vi "4DOF_Serial_Write_Read_Event_xbox_Polling.vi"() -> ()   [LabVIEW 2023]
uses:
  <vilib>/MakerHub/Xbox-One-Controller/Private/Type Defs/Indicators/Controller.ctl
  <vilib>/MakerHub/Xbox-One-Controller/Private/Type Defs/Indicators/A.ctl
  <vilib>/MakerHub/Xbox-One-Controller/Private/Type Defs/Indicators/B.ctl
  <vilib>/MakerHub/Xbox-One-Controller/Private/Type Defs/Indicators/X.ctl
  <vilib>/MakerHub/Xbox-One-Controller/Private/Type Defs/Indicators/Y.ctl
  <vilib>/MakerHub/Xbox-One-Controller/Private/Type Defs/Indicators/Left Bumper.ctl
  <vilib>/MakerHub/Xbox-One-Controller/Private/Type Defs/Indicators/Right Bumper.ctl
  <vilib>/MakerHub/Xbox-One-Controller/Private/Type Defs/Indicators/View.ctl
  <vilib>/MakerHub/Xbox-One-Controller/Private/Type Defs/Indicators/Menu.ctl
  <vilib>/MakerHub/Xbox-One-Controller/Private/Type Defs/Indicators/Thumbstick_Analog.ctl
  <vilib>/MakerHub/Xbox-One-Controller/Private/Type Defs/Indicators/Slider.ctl
  <vilib>/MakerHub/Xbox-One-Controller/Private/Type Defs/Indicators/DPad.ctl
  <vilib>/MakerHub/Xbox-One-Controller/Public/Open First Controller.vi
  <vilib>/Instr/_visa.llb/VISA Configure Serial Port (Instr).vi
  <vilib>/MakerHub/Xbox-One-Controller/LMH-Xbox-One-Controller.lvlib
panel:
  in  "?":bool
  in  "?":bool
  out "length":i32
  out "IK Cartesian \nCordinates (mm)\nLast Sent":string
  in  "Enter IK (X/Y/Z)":string[](array[string])
  in  "Refresh Buffer":bool
  out "X Axis Right":i32 format="%#.0f"
  out "Y Axis Left":i32
  out "Error Out":errorcluster
  in  "byte count\nRead":u32=80
  out "Serial Buffer (Read)":string
  in  "Left Stick":u32(slide)=50 scale=0.0..100.0
  out "Loop Count":i32
  out "Panel Controls\nActive":bool
  in  "Right Bumper":T1 caption="Blank Button"
  in  "Left Bumper":T2 caption="Blank Button"
  in  "Jog\nS_Joint_State\nVia Manual Jog":T3 caption="Blank Button"
  in  "Jog\nS_Main_System_State":T4 caption="Blank Button"
  in  "Home J4":T5 caption="Blank Button"
  in  "Home J2":T6 caption="Blank Button"
  in  "Home J3":T7 caption="Blank Button"
  in  "Home J1":T8 caption="Blank Button"
  in  "Right Stick":u32(slide)=50 scale=0.1..100.0
  in  "Panel Buttons / Xbox Buttons":bool
  out "Controller":T9={"A Button"=FALSE, "B Button"=FALSE, "X Button"=FALSE, "Y Button"=FALSE, "Left Bumper"=FALSE, "Right Bumper"=FALSE, "View Button"=FALSE, "Menu Button"=FALSE, "Left Stick"={[], []}, "Right Stick"={[], []}, "Trigger"=0, "D-Pad"=5} {"Trigger" scale=32767.0..-32768.0}
  out "error out":errorcluster
  in  "error in (no error)":errorcluster
  in  "Loop Timer ms":u32=5 min=10
  out "Concatenated \nString For Transmission":string
  in  "VISA resource name":refnum<visa-resource-name>="COM8"
  out "byte count \nSent":u32
  out "Controller Outputs\nActive":bool
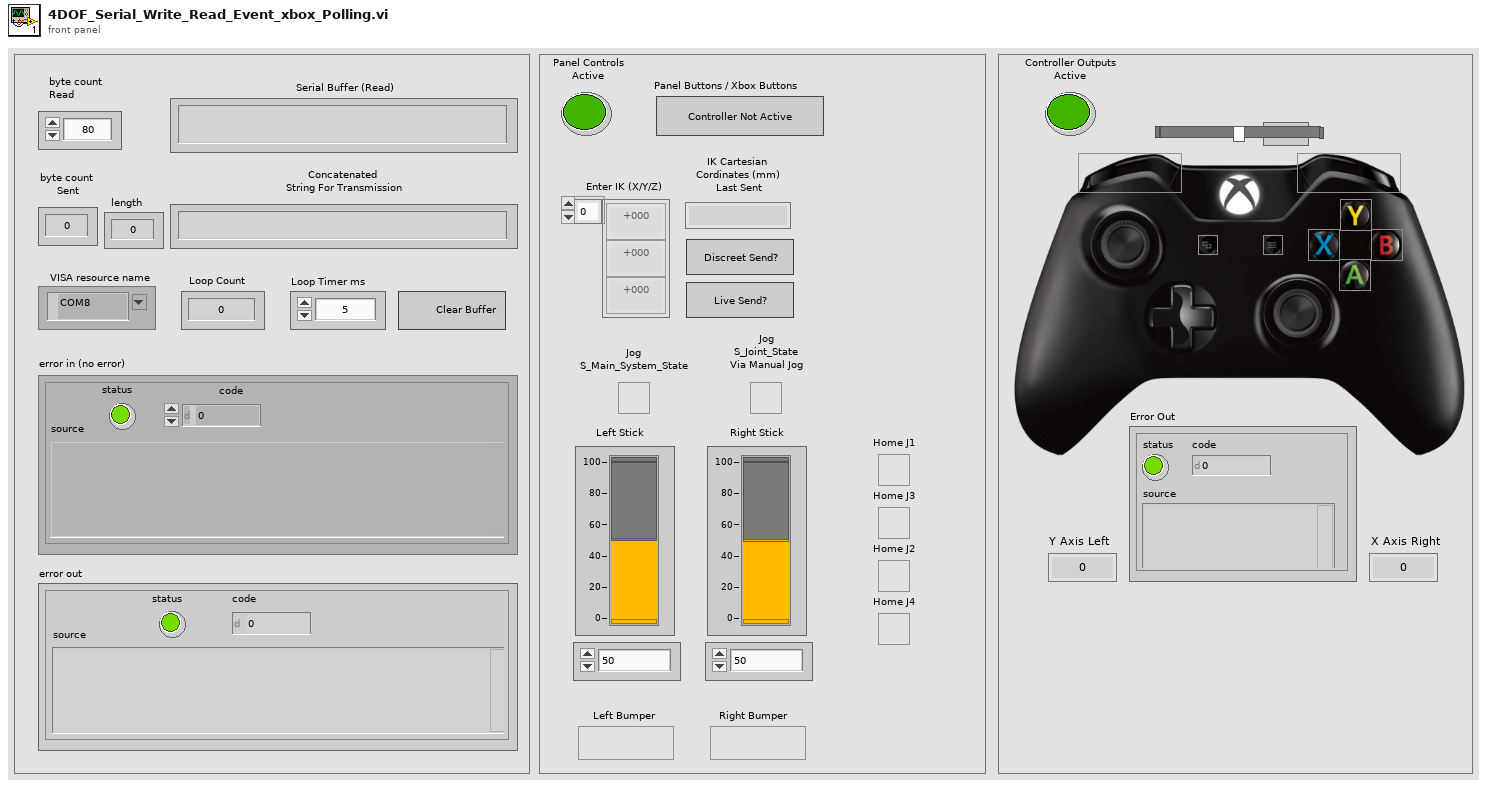
[diagram p1: front panel]
types:
  T1 = typedef "LMH-Xbox-One-Controller.lvlib/Right Bumper.ctl" = bool
  T2 = typedef "LMH-Xbox-One-Controller.lvlib/Left Bumper.ctl" = bool
  T3 = typedef "LMH-Xbox-One-Controller.lvlib/Menu.ctl" = bool
  T4 = typedef "LMH-Xbox-One-Controller.lvlib/View.ctl" = bool
  T5 = typedef "LMH-Xbox-One-Controller.lvlib/Y.ctl" = bool
  T6 = typedef "LMH-Xbox-One-Controller.lvlib/X.ctl" = bool
  T7 = typedef "LMH-Xbox-One-Controller.lvlib/B.ctl" = bool
  T8 = typedef "LMH-Xbox-One-Controller.lvlib/A.ctl" = bool
  T9 = typedef "LMH-Xbox-One-Controller.lvlib/Controller.ctl" = cluster{"A Button":T8, "B Button":T7, "X Button":T6, "Y Button":T5, "Left Bumper":T2, "Right Bumper":T1, "View Button":T4, "Menu Button":T3, "Left Stick":T10, "Right Stick":T10, "Trigger":T11, "D-Pad":T12}
  T10 = typedef "LMH-Xbox-One-Controller.lvlib/Thumbstick_Analog.ctl" = cluster{i32[], i32[]}
  T11 = typedef "LMH-Xbox-One-Controller.lvlib/Slider.ctl" = i32
  T12 = typedef "LMH-Xbox-One-Controller.lvlib/DPad.ctl" = u16
  T13 = typedef "LMH-Xbox-One-Controller.lvlib/Xbox One Controller Ref.ctl" = cluster{"Controller Ref":refnum<k1>, "Event Refnum":refnum<event-registration>, "Worker Ref":refnum<vi>}
  T14 = typedef "LMH-Xbox-One-Controller.lvlib/All Axis Data.ctl" = cluster{"Left Stick":cluster{"X Axis":i32, "Y Axis":i32}, "Right Stick":cluster{"X Axis":i32, "Y Axis":i32}, "Triggers":i32, "D-Pad":T15}
  T15 = typedef "LMH-Xbox-One-Controller.lvlib/DPad Enum.ctl" = enum16{"Idle", "Up", "Up / Right", "Right", "Down / Right", "Down", "Down / Left", "Left", "Up / Left"}
  T16 = typedef "LMH-Xbox-One-Controller.lvlib/All Buttons Visual.ctl" = cluster{"A":T8, "B":T7, "X":T6, "Y":T5, "Left Bumper":T2, "Right Bumper":T1, "View Button":T4, "Menu Button":T3, "Left Stick":T17, "Right Stick":T17}
  T17 = typedef "LMH-Xbox-One-Controller.lvlib/Thumbstick.ctl" = bool
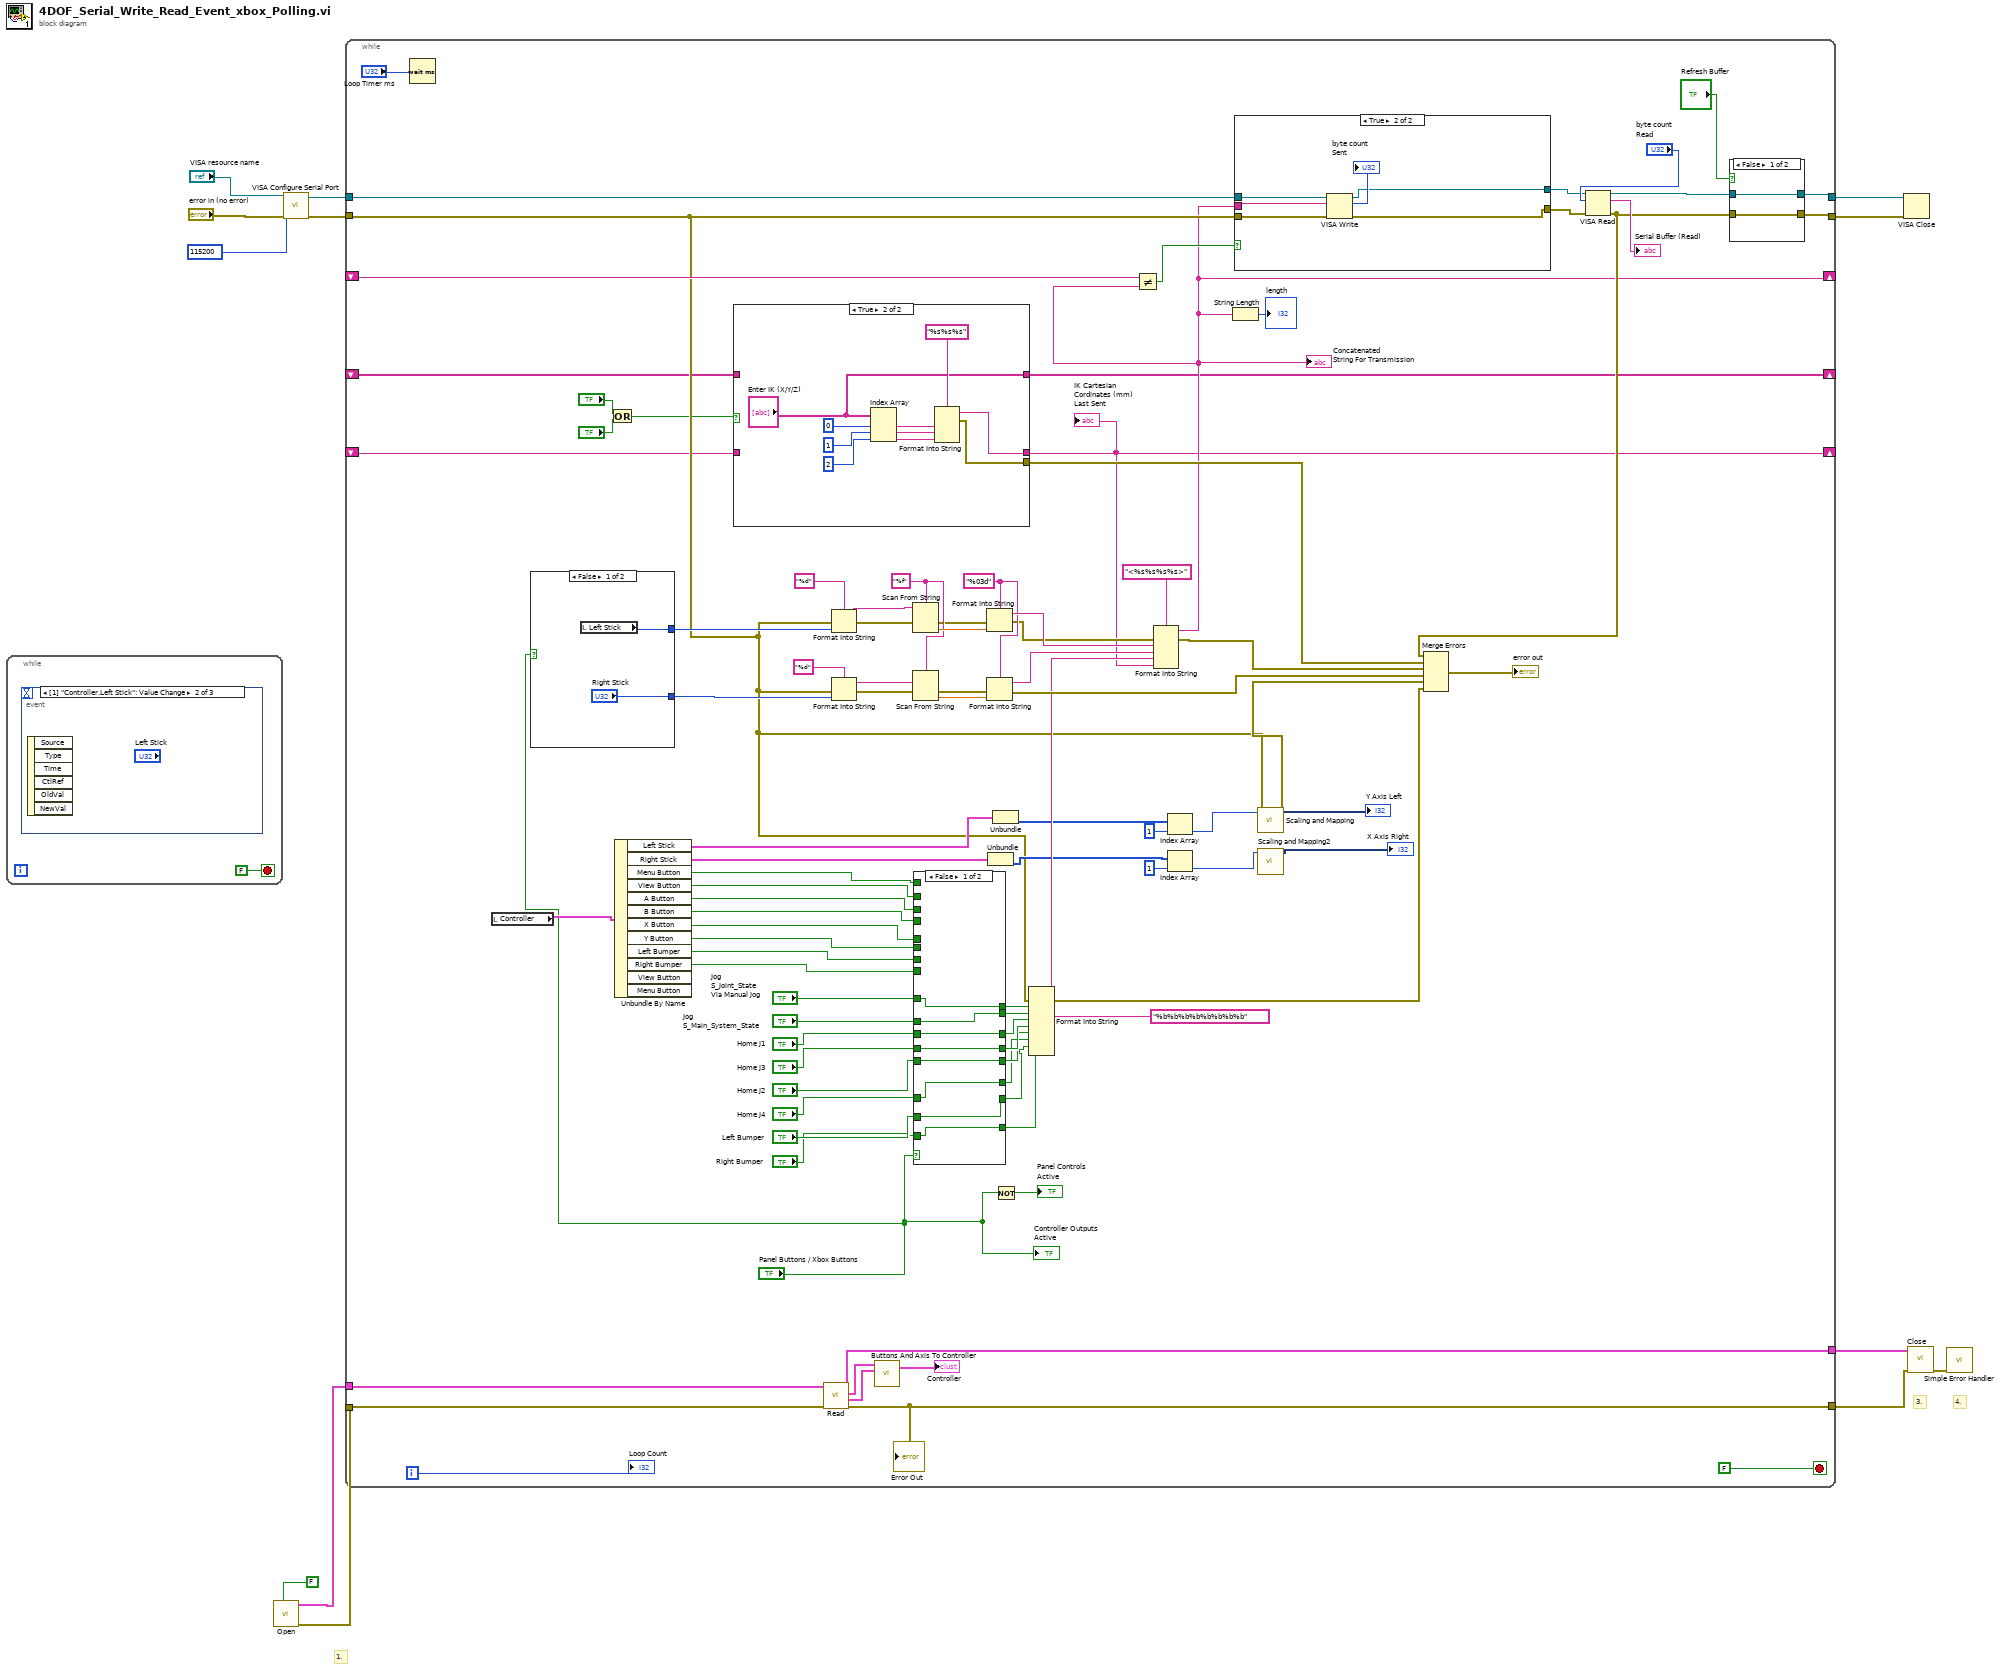
[diagram p0: block diagram]
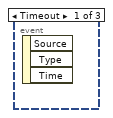
[diagram p2: hidden frame]
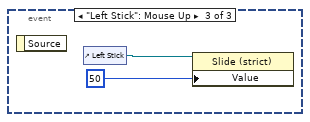
[diagram p3: hidden frame]
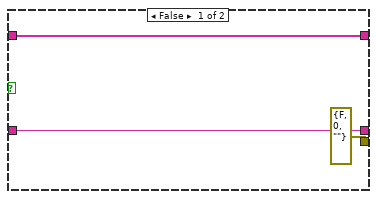
[diagram p4: hidden frame]
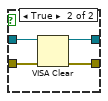
[diagram p5: hidden frame]
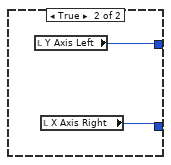
[diagram p6: hidden frame]
diagram:
  # "4."
  # "3."
  # "1."
  n1 = while {
    stop <- FALSE stop-if-true
    n2 = event shown="[1] \"Controller.Left Stick\": Value Change" {
      selector: _ -> [_ _ _]
      dyn-events: _ -> [_ _ _]
      timeout: _ -> [_ _ _]
      event Timeout {
        n3 = event-data() -> ()  [unwired: 1 in, 3 out]
      }
      event Value Change {
        n4 = event-data() -> ()  [unwired: 1 in, 6 out]
      }
      event "Left Stick": Mouse Up {
        n5 = event-data() -> ()  [unwired: 1 in, 1 out]
        n6 = control-ref of="Left Stick"() -> (w16:refnum<vi>)
        n7 = property class="Slide (strict)"(reference=w16, "Value"=u32 50) -> ()  [unwired: 1 in, 2 out]
      }
    }
  }
  n8 = call-poly <vilib>:"Open.vi"("Enable Events (T)"=FALSE) -> ("Error Out"=w4:errorcluster, "Xbox One Controller"=w5:T13)  [unwired: 8 in, 1 out]
  n9 = call-poly "VISA Configure Serial Port"("VISA resource name"="VISA resource name", "baud rate (9600)"=u32 115200, "error in (no error)"="error in (no error)") -> ("VISA resource name out"=w6:refnum<visa-resource-name>, "error out"=w1:errorcluster)  [unwired: 11 in]
  n10 = while {
    tunnel: w1 -> [w28]
    tunnel: [w30] -> w8
    tunnel: [w31] -> w7
    tunnel: w6 -> [w52]
    shift-right: [w25] -> _
    shift-left: _ -> [w54]
    tunnel: w5 -> [w48]
    tunnel: w4 -> [w47]
    tunnel: [w46] -> w3
    tunnel: [w45] -> w2
    shift-right: [w23] -> _
    shift-left: _ -> [w22]
    shift-right: [w21] -> _
    shift-left: _ -> [w20]
    i -> [w60]
    stop <- FALSE stop-if-true
    w104 = "%f" ("format string")
    w106 = "%03d" ("format string")
    n11 = Wait (ms)(milliseconds to wait="Loop Timer ms") -> ()  [unwired: 1 out]
    n12 = local read "Controller"() -> (w59:T9)
    n13 = case shown="False" "Panel Buttons / Xbox Buttons" {
      tunnel: ["Right Stick" w133] -> w62
      tunnel: [w131 w134] -> w56
      frame False {
        n14 = local read "Left Stick"() -> (w131:u32)
      }
      frame True {
        n15 = local read "Y Axis Left"() -> (w134:i32)
        n16 = local read "X Axis Right"() -> (w133:i32)
      }
    }
    n17 = Or(x="?", y="?") -> (x .or. y?=w17:bool)
    n18 = Unbundle By Name(w59) -> ("Left Stick"=w92:T10, "Right Stick"=w91:T10, "Menu Button"=w70:T3, "View Button"=w69:T4, "A Button"=w68:T8, "B Button"=w67:T7, "X Button"=w66:T6, "Y Button"=w65:T5, "Left Bumper"=w64:T2, "Right Bumper"=w63:T1)  [unwired: 2 out]
    n19 = case shown="True" w17 {
      tunnel: [w113 w117] -> w21
      tunnel: [errorcluster {"status"=FALSE, "code"=0, "source"=""} ("error IO") w116] -> w26
      tunnel: [w114 "Enter IK (X/Y/Z)"] -> w23
      tunnel: w22 -> [w114 _]
      tunnel: w20 -> [w113 _]
      frame False {
      }
      frame True {
        n20 = Index Array(array="Enter IK (X/Y/Z)", index #1=0 ("index"), index #2=1 ("index"), index #3=2 ("index")) -> (element #1=w121:string, element #2=w120:string, element #3=w119:string)
        n21 = Format Into String(format string="%s%s%s", w121, w120, w119) -> (resulting string=w117:string, error out=w116:errorcluster)  [unwired: 2 in]
      }
    }
    "IK Cartesian \nCordinates (mm)\nLast Sent" <- w21
    n22 = call <vilib>:"Read.vi"("Error In"=w47, "Xbox One Controller Ref"=w48) -> ("Error Out"=w46:errorcluster, "All Axis"=w50:T14, "Buttons"=w49:T16, "Xbox One Controller Ref"=w45:T13)  [unwired: 6 in]
    "Error Out" <- w46
    n23 = Format Into String(format string="%d", error in=w28, w56) -> (resulting string=w110:string, error out=w100:errorcluster)  [unwired: 1 in]
    n24 = Format Into String(format string="%d", error in=w28, w62) -> (resulting string=w105:string, error out=w97:errorcluster)  [unwired: 1 in]
    n25 = call <vilib>:"Buttons And Axis To Controller.vi"("All Axis"=w50, "Buttons"=w49) -> ("Controller"=→"Controller":T9)  [unwired: 5 in]
    n26 = Scan From String(format string=w104, input string=w110, error in=w100) -> (error out=w99:errorcluster, output 1=w111:dbl)  [unwired: 2 in, 2 out]
    n27 = Scan From String(format string=w104, input string=w105, error in=w97) -> (error out=w96:errorcluster, output 1=w101:dbl)  [unwired: 2 in, 2 out]
    n28 = case shown="False" "Panel Buttons / Xbox Buttons" {
      tunnel: "Jog\nS_Joint_State\nVia Manual Jog" -> [w150 _]
      tunnel: [w150 w158] -> w85
      tunnel: "Jog\nS_Main_System_State" -> [w149 _]
      tunnel: [w149 w157] -> w83
      tunnel: "Home J1" -> [w148 _]
      tunnel: [w148 w156] -> w81
      tunnel: "Home J3" -> [w147 _]
      tunnel: "Home J2" -> [w146 _]
      tunnel: "Home J4" -> [w145 _]
      tunnel: "Left Bumper" -> [w144 _]
      tunnel: "Right Bumper" -> [w143 _]
      tunnel: [w147 w155] -> w75
      tunnel: [w146 w154] -> w74
      tunnel: [w145 w153] -> w73
      tunnel: [w144 w152] -> w72
      tunnel: [w143 w151] -> w71
      tunnel: w70 -> [_ w158]
      tunnel: w69 -> [_ w157]
      tunnel: w68 -> [_ w156]
      tunnel: w67 -> [_ w155]
      tunnel: w66 -> [_ w154]
      tunnel: w65 -> [_ w153]
      tunnel: w64 -> [_ w152]
      tunnel: w63 -> [_ w151]
      frame False {
      }
      frame True {
      }
    }
    n29 = Format Into String(format string=w106, error in=w99, w111) -> (resulting string=w109:string, error out=w98:errorcluster)  [unwired: 1 in]
    n30 = Format Into String(format string=w106, error in=w96, w101) -> (resulting string=w107:string, error out=w94:errorcluster)  [unwired: 1 in]
    n31 = Unbundle(w91) -> (w41:i32[])  [unwired: 1 out]
    n32 = Unbundle(w92) -> (w44:i32[])  [unwired: 1 out]
    n33 = Not(x="Panel Buttons / Xbox Buttons") -> (.not. x?=→"Panel Controls\nActive":bool)
    n34 = Format Into String(format string="%b%b%b%b%b%b%b%b", error in=w28, w85, w83, w81, w75, w74, w73, w72, w71) -> (resulting string=w88:string, error out=w61:errorcluster)  [unwired: 1 in]
    n35 = Format Into String(format string="<%s%s%s%s>", error in=w98, w109, w107, w88, w21) -> (resulting string=w25:string, error out=w95:errorcluster)  [unwired: 1 in]
    "Concatenated \nString For Transmission" <- w25
    n36 = Not Equal?(x=w54, y=w25) -> (x != y?=w53:bool)
    n37 = Index Array(array=w44, index=1) -> (element=w42:i32)
    n38 = Index Array(array=w41, index=1) -> (element=w39:i32)
    n39 = String Length(string=w25) -> (length=→"length":i32)
    n40 = case shown="True" w53 {
      tunnel: w28 -> [w135 w141]
      tunnel: w52 -> [w136 w140]
      tunnel: w25 -> [_ w139]
      tunnel: [w135 w138] -> w36
      tunnel: [w136 w137] -> w34
      frame False {
      }
      frame True {
        n41 = VISA Write(VISA resource name=w140, write buffer=w139, error in (no error)=w141) -> (VISA resource name out=w137:refnum<visa-resource-name>, return count=→"byte count \nSent":u32, error out=w138:errorcluster)
      }
    }
    n42 = call "Scaling and Mapping"("error in (no error)"=w28, "Signals"=w42) -> ("error out"=w89:errorcluster, "Scaled Signals"=→"Y Axis Left":dynamicdata)  [unwired: 8 in]
    n43 = call "Scaling and Mapping2"("Signals"=w39) -> ("Scaled Signals"=→"X Axis Right":dynamicdata)  [unwired: 9 in, 1 out]
    n44 = VISA Read(VISA resource name=w34, byte count="byte count\nRead", error in (no error)=w36) -> (VISA resource name out=w32:refnum<visa-resource-name>, read buffer=→"Serial Buffer (Read)":string, error out=w27:errorcluster)  [unwired: 1 out]
    n45 = Merge Errors(w27, w26, w95, w94, w89, w61) -> (→"error out":errorcluster)
    n46 = case shown="False" "Refresh Buffer" {
      tunnel: w32 -> [w126 w130]
      tunnel: w27 -> [w125 w129]
      tunnel: [w126 w128] -> w31
      tunnel: [w125 w127] -> w30
      frame False {
      }
      frame True {
        n47 = VISA Clear(VISA resource name=w130, error in (no error)=w129) -> (VISA resource name out=w128:refnum<visa-resource-name>, error out=w127:errorcluster)
      }
    }
    "Controller Outputs\nActive" <- "Panel Buttons / Xbox Buttons"
    "Loop Count" <- w60
  }
  n48 = VISA Close(VISA resource name=w7, error in (no error)=w8) -> ()  [unwired: 1 out]
  n49 = call <vilib>:"Close.vi"("Error In"=w3, "Xbox One Controller Ref"=w2) -> ("Error Out"=w11:errorcluster)  [unwired: 9 in]
  n50 = call <vilib>:"Simple Error Handler.vi"("error in (no error)"=w11) -> ()  [unwired: 4 in, 5 out]
